vi "Dynamic Lock 1k.vi"(9 "Page Selection":T1=enum."E0-E1 [13]", 11 "PN532 COM Port":refnum<visa-resource-name>) -> (0 "Error out":errorcluster, 2 "Succeeded":bool, 3 "PN532 COM Port Out":refnum<visa-resource-name>)   [LabVIEW 2012, in "NFC Driver.lvlib"]
uses:
  NFC Driver.lvlib
  Typedef/Dynamic Lock Page Section 1K.ctl
panel:
  out "result string":string
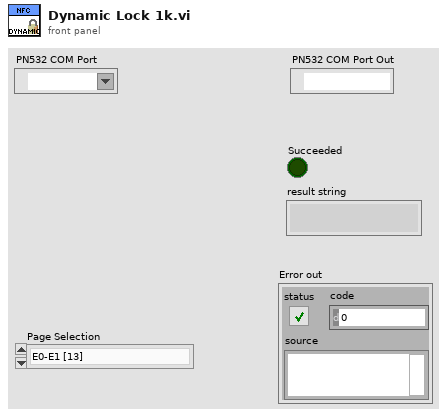
[diagram p1: front panel]
types:
  T1 = typedef "NFC Driver.lvlib/Dynamic Lock Page Section 1K.ctl" = enum16{"10-1F [0]", "20-2F [1]", "30-3F [2]", "40-4F [3]", "50-5F [4]", "60-6F [5]", "70-7F [6]", "80-8F [7]", "90-9F [8]", "A0-AF [9]", "B0-BF [10]", "C0-CF [11]", "D0-DF [12]", "E0-E1 [13]"}
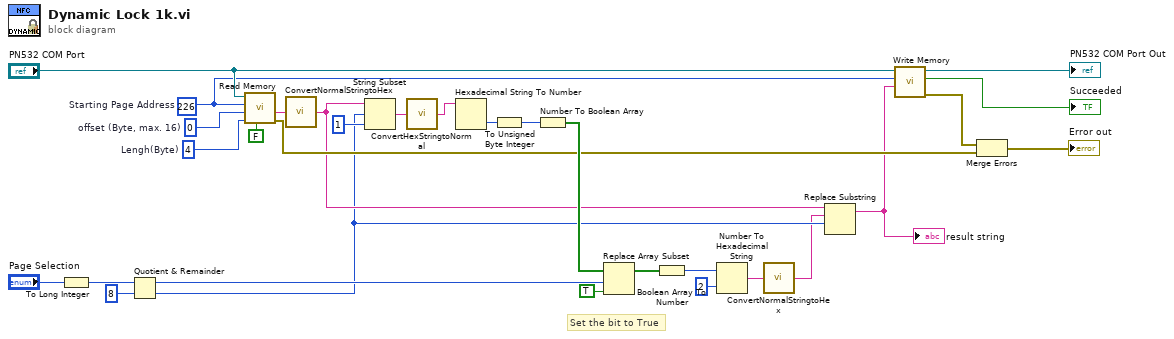
[diagram p0: block diagram]
diagram:
  w10 = 0  # offset (Byte, max. 16)
  w28 = 4  # Lengh(Byte)
  w8 = 226  # Starting Page Address
  # "Set the bit to True"
  n1 = To Long Integer(number="Page Selection") -> (32bit integer=w17:i32)
  n2 = Quotient & Remainder(x=w17, y=8) -> (x-y*floor(x/y)=w18:i32, floor(x/y)=w7:i32)
  n3 = call "Read Memory.vi"("Reverse Output[F]"=FALSE, "length (Byte, max. 16)"=w28, "offset (Byte, max. 16)"=w10, "Page Address"=w8, "PN532 COM Port"="PN532 COM Port") -> ("error out"=w22:errorcluster, "Selected substring (HEX)"=w1:string)  [unwired: 2 in, 3 out]
  n4 = call "ConvertNormalStringtoHex.vi"("Normal String"=w1) -> ("Hex String"=w9:string)
  n5 = String Subset(string=w9, offset (0)=w7, length (rest)=1 ("length (rest)")) -> (substring=w14:string)
  n6 = call "ConvertHexStringtoNormal.vi"("Hex String"=w14) -> ("Normal String"=w13:string)
  n7 = Hexadecimal String To Number(string=w13) -> (number=w27:u32)  [unwired: 2 in, 1 out]
  n8 = To Unsigned Byte Integer(number=w27) -> (unsigned 8bit integer=w15:u8)
  n9 = Number To Boolean Array(number=w15) -> (Boolean array=w26:bool[])
  n10 = Replace Array Subset(array=w26, new element=TRUE ("new element/subarray"), index=w18) -> (w21:bool[])
  n11 = Boolean Array To Number(Boolean array=w21) -> (number=w25:u32)
  n12 = Number To Hexadecimal String(1:i16 2 ("width (-)"), 2:w25) -> (0:w6:string)
  n13 = call "ConvertNormalStringtoHex.vi"("Normal String"=w6) -> ("Hex String"=w4:string)
  n14 = Replace Substring(3:w7, 4:w4, 5:w9) -> (1:w5:string)  [unwired: 1 in, 1 out]
  "result string" <- w5
  n15 = call "Write Memory.vi"("Data to write (HEX, max 16 bytes)"=w5, "Page Address"=w8, "PN532 COM Port"="PN532 COM Port") -> ("Error Out"=w23:errorcluster, "Succesful?"=→"Succeeded":bool, "PN532 COM Port Out"=→"PN532 COM Port Out":refnum<visa-resource-name>)  [unwired: 6 in]
  n16 = Merge Errors(w23, w22) -> (→"Error out":errorcluster)
